vi "LocalizationFGV.vi"(0 "Action":T1, 1 "Dictionary File Path":path, 5 "VI in":refnum<vi>, 7 "Target Language":string, 9 "UID":string, 11 "error in":errorcluster) -> (6 "Dictionary":T2, 8 "Languages":string[](array[string]), 10 "Translated Word":string, 14 "Current Language":string, 15 "error out":errorcluster)   [LabVIEW 2017, in "JKI Simple Localization.lvlib"]
uses:
  API/JKI Simple Localization.lvlib
  Definitions/Dictionary--Cluster.ctl
  Definitions/Private/Font -- Cluster.ctl
  Definitions/Private/Phrase Dictionary Entry -- Cluster.ctl
  Definitions/Private/Localization FGV Action -- Enum.ctl
  Definitions/Private/VI Info -- Cluster.ctl
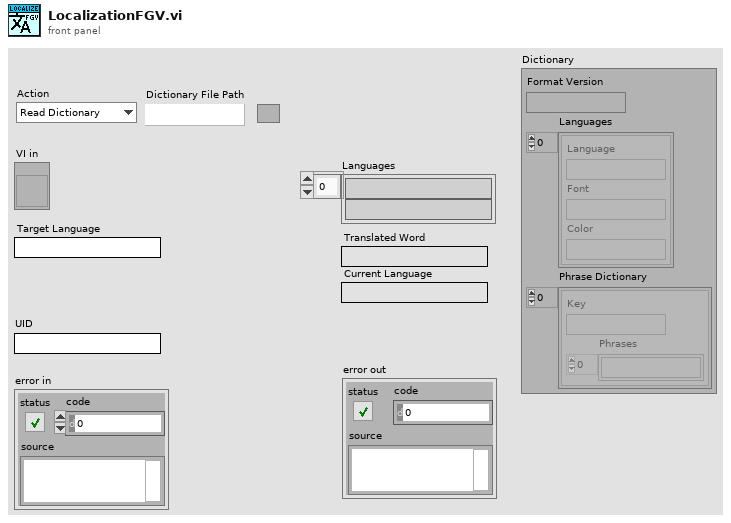
[diagram p1: front panel]
types:
  T1 = typedef "JKI Simple Localization.lvlib/Localization FGV Action -- Enum.ctl" = enum16{"Read Dictionary", "Translate VIs", "Register VI", "Get Languages", "Translate Phrase", "Translate VI", "Unregister"}
  T2 = typedef "JKI Simple Localization.lvlib/Dictionary--Cluster.ctl" = cluster{"Format Version":string, "Languages":T3[], "Phrase Dictionary":T4[]}
  T3 = typedef "JKI Simple Localization.lvlib/Font -- Cluster.ctl" = cluster{"Language":string, "Font":string, "Color":string}
  T4 = typedef "JKI Simple Localization.lvlib/Phrase Dictionary Entry -- Cluster.ctl" = cluster{"Key":string, "Phrases":string[]}
  T5 = typedef "JKI Simple Localization.lvlib/VI Info -- Cluster.ctl" = cluster{"VI Ref":refnum<vi>, "Language":string}
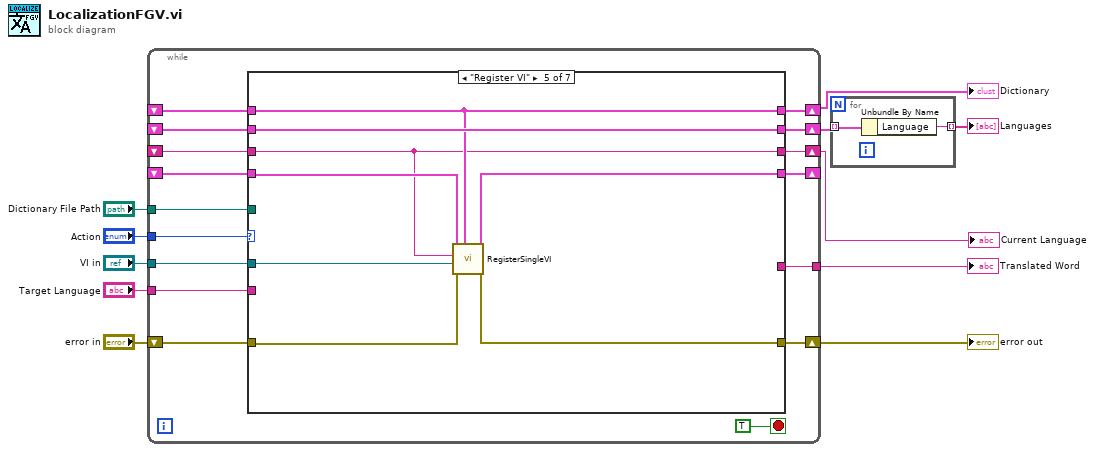
[diagram p0: block diagram]
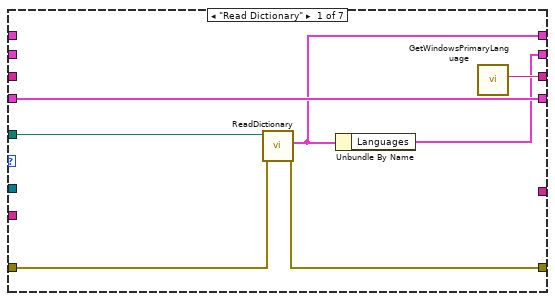
[diagram p2: hidden frame]
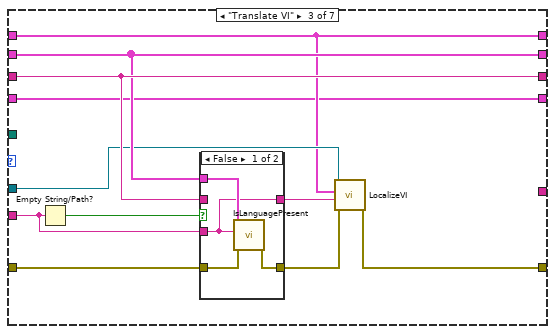
[diagram p4: hidden frame]
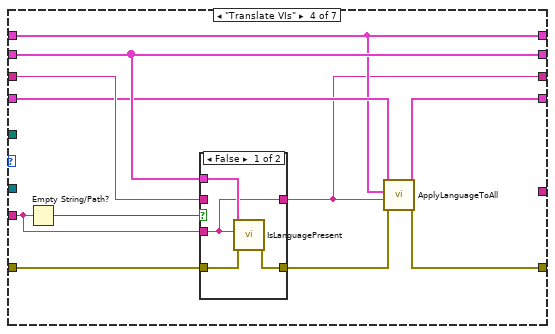
[diagram p6: hidden frame]
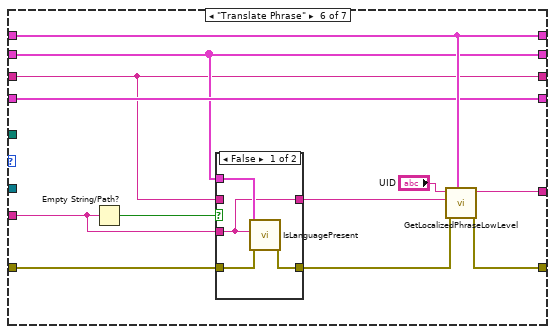
[diagram p8: hidden frame]
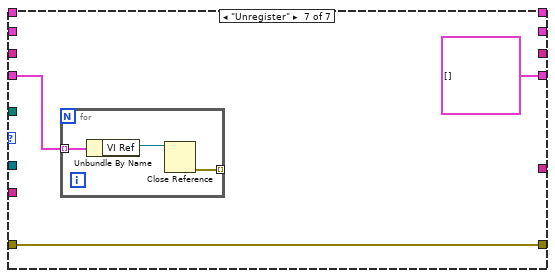
[diagram p10: hidden frame]
diagram:
  n1 = while {
    tunnel: "Action" -> [w26]
    tunnel: "Dictionary File Path" -> [w25]
    shift-right: [w24] -> w3
    shift-left: _ -> [w23]
    shift-right: [w13] -> w10
    shift-left: "error in" -> [w22]
    tunnel: "VI in" -> [w21]
    shift-right: [w20] -> _
    shift-left: _ -> [w19]
    shift-right: [w18] -> w2
    shift-left: _ -> [w17]
    tunnel: "Target Language" -> [w16]
    shift-right: [w15] -> w4
    shift-left: _ -> [w14]
    tunnel: [w12] -> w6
    stop <- TRUE stop-if-true
    n2 = case shown="\"Register VI\"" w26 {
      tunnel: w25 -> [w34 _ _ _ _ _ _]
      tunnel: [w29 w39 w42 w60 w78 w93 _] -> w24
      tunnel: w23 -> [_ w39 w42 w60 w78 w93 _]
      tunnel: w22 -> [w32 w36 w46 w63 w80 w88 w102]
      tunnel: w21 -> [_ _ w43 _ w74 _ _]
      tunnel: [w31 w37 w40 w61 w76 w91 T5[] [] ("VI Status")] -> w20
      tunnel: w19 -> [w31 w37 w40 w62 w77 w91 w101]
      tunnel: [w28 w38 w47 w64 w81 w86 _] -> w18
      tunnel: w17 -> [_ w38 w47 w64 w81 w86 _]
      tunnel: w16 -> [_ _ w48 w65 _ w84 _]
      tunnel: [w30 w35 w49 w57 w75 w83 _] -> w15
      tunnel: w14 -> [_ w35 w49 w66 w75 w83 _]
      tunnel: [w33 w36 w44 w58 w79 w92 w102] -> w13
      tunnel: [_ _ _ _ _ w90 _] -> w12
      frame "Read Dictionary" {
        n3 = call "ReadDictionary.vi"("error in (no error)"=w32, "Dictionary File Path"=w34) -> ("error out"=w33:errorcluster, "Dictionary"=w29:T2)  [unwired: 6 in, 2 out]
        n4 = Unbundle By Name(w29) -> ("Languages"=w28:T3[])
        n5 = call "GetWindowsPrimaryLanguage.vi"() -> ("Primary Language"=w30:string)  [unwired: 11 in]
      }
      frame "Get Languages" {
      }
      frame "Translate VI" {
        n6 = Empty String/Path?(string/path=w48) -> (empty?=w50:bool)
        n7 = case shown="False" w50 {
          tunnel: [w52 w55] -> w41
          tunnel: w49 -> [_ w55]
          tunnel: w48 -> [w52 _]
          tunnel: w47 -> [w54 _]
          tunnel: w46 -> [w53 w56]
          tunnel: [w51 w56] -> w45
          frame False {
            n8 = call "IsLanguagePresent.vi"("error in"=w53, "Target Language"=w52, "Languages"=w54) -> ("error out"=w51:errorcluster)  [unwired: 7 in, 1 out]
          }
          frame True {
          }
        }
        n9 = call "LocalizeVI.vi"("error in (no error)"=w45, "Target Language"=w41, "Dictionary"=w42, "VI in"=w43) -> ("error out"=w44:errorcluster)  [unwired: 7 in]
      }
      frame "Translate VIs" {
        n10 = Empty String/Path?(string/path=w65) -> (empty?=w67:bool)
        n11 = case shown="False" w67 {
          tunnel: [w69 w72] -> w57
          tunnel: w66 -> [_ w72]
          tunnel: w65 -> [w69 _]
          tunnel: w64 -> [w71 _]
          tunnel: w63 -> [w70 w73]
          tunnel: [w68 w73] -> w59
          frame False {
            n12 = call "IsLanguagePresent.vi"("error in"=w70, "Target Language"=w69, "Languages"=w71) -> ("error out"=w68:errorcluster)  [unwired: 7 in, 1 out]
          }
          frame True {
          }
        }
        n13 = call "ApplyLanguageToAll.vi"("error in (no error)"=w59, "Target Language"=w57, "Dictionary"=w60, "VI Status"=w62) -> ("error out"=w58:errorcluster, "VI Status"=w61:T5[])  [unwired: 6 in]
      }
      frame "Register VI" {
        n14 = call "RegisterSingleVI.vi"("Dictionary"=w78, "error in (no error)"=w80, "VI in"=w74, "Target Language"=w75, "VI Status"=w77) -> ("Error out"=w79:errorcluster, "VI Status"=w76:T5[])  [unwired: 5 in]
      }
      frame "Translate Phrase" {
        n15 = Empty String/Path?(string/path=w84) -> (empty?=w85:bool)
        n16 = case shown="False" w85 {
          tunnel: [w95 w98] -> w82
          tunnel: w83 -> [_ w98]
          tunnel: w84 -> [w95 _]
          tunnel: w86 -> [w97 _]
          tunnel: w88 -> [w96 w99]
          tunnel: [w94 w99] -> w87
          frame False {
            n17 = call "IsLanguagePresent.vi"("error in"=w96, "Target Language"=w95, "Languages"=w97) -> ("error out"=w94:errorcluster)  [unwired: 7 in, 1 out]
          }
          frame True {
          }
        }
        n18 = call "GetLocalizedPhraseLowLevel.vi"("Dictionary"=w93, "error in (no error)"=w87, "Target Language"=w82, "Key"="UID") -> ("error out"=w92:errorcluster, "Localized Phrase"=w90:string)  [unwired: 6 in]
      }
      frame "Unregister" {
        n19 = for {
          tunnel: w101 -> [w105] mode=indexing
          tunnel: [w103] -> _ mode=indexing
          n20 = Unbundle By Name(w105) -> ("VI Ref"=w104:refnum<vi>)
          n21 = Close Reference(reference=w104) -> (error out=w103:errorcluster)  [unwired: 1 in]
        }
      }
    }
  }
  "error out" <- w10
  "Dictionary" <- w3
  "Translated Word" <- w6
  "Current Language" <- w4
  n22 = for {
    tunnel: w2 -> [w107] mode=indexing
    tunnel: [w106] -> w1 mode=indexing
    n23 = Unbundle By Name(w107) -> ("Language"=w106:string)
  }
  "Languages" <- w1
